vi "moduleGet.vi"() -> ()   [LabVIEW 2020]
uses:
  <vilib>/Rock Robotics/WPI/ThirdParty/JAS_Junk/TrajLib/Trajectory_Library.lvlib
panel:
  in  "p":bool
  in  "Distance":dbl
  in  "angle":dbl
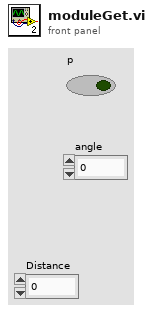
[diagram p1: front panel]
types:
  T1 = typedef "Trajectory_Library.lvlib/ROTATION2D.ctl" = cluster{"VALUE":dbl, "COS":dbl, "SIN":dbl}
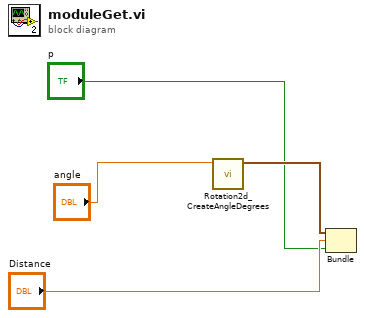
[diagram p0: block diagram]
diagram:
  n1 = call <vilib>:"Rotation2d_CreateAngleDegrees.vi"("Angle_Degrees"="angle") -> ("ROTATION"=w3:T1)  [unwired: 10 in]
  n2 = Bundle("ROTATION"=w3, "Distance"="Distance", "p"="p") -> (w4:cluster{"ROTATION":T1, "Distance":dbl, "p":bool})  [unwired: 1 in]
